vi "Main.vi"() -> ()   [LabVIEW 2017]
uses:
  <vilib>/LAVA/UI Tools/Fading/_Fade In(I32)__lava_lib_ui_tools.vi
  <vilib>/LAVA/UI Tools/Fading/_Fade Out(I32)__lava_lib_ui_tools.vi
panel:
  out "date string":string
  out "time string":string
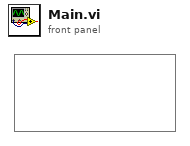
[diagram p1: front panel]
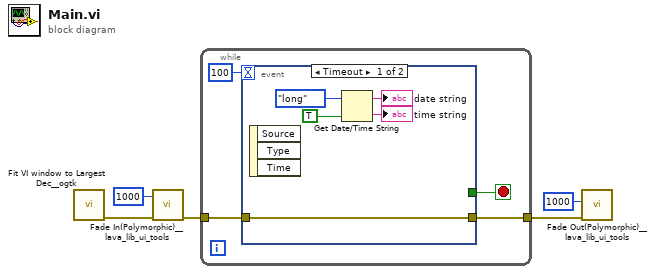
[diagram p0: block diagram]
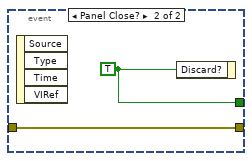
[diagram p2: hidden frame]
diagram:
  n1 = call <userlib>:"Fit VI window to Largest Dec__ogtk.vi"() -> ("error out"=w5:errorcluster)  [unwired: 6 in, 1 out]
  n2 = call-poly <vilib>:"Fade In(Polymorphic)__lava_lib_ui_tools.vi"("error in"=w5, "Fade time (ms)"=1000) -> ("error out"=w4:errorcluster)  [unwired: 8 in, 1 out]
  n3 = while {
    tunnel: w4 -> [w7]
    tunnel: [w6] -> w3
    stop <- w9 stop-if-true
    n4 = event shown="[0] Timeout" {
      selector: _ -> [_ _]
      dyn-events: _ -> [_ _]
      timeout: 100 -> [_ _]
      tunnel: [_ w16] -> w9
      tunnel: w7 -> [w10 w15]
      tunnel: [w10 w15] -> w6
      event Timeout {
        n5 = event-data() -> ()  [unwired: 1 in, 3 out]
        n6 = Get Date/Time String(date format (0)=enum16{"short", "long", "abbreviated"}."long", want seconds? (F)=TRUE) -> (date string=→"date string":string, time string=→"time string":string)  [unwired: 1 in]
      }
      event Panel Close? {
        w16 = TRUE ("Discard?")
        n7 = event-data() -> ()  [unwired: 1 in, 4 out]
        n8 = event-data("Discard?"=w16) -> ()  [unwired: 1 in, 1 out]
      }
    }
  }
  n9 = call-poly <vilib>:"Fade Out(Polymorphic)__lava_lib_ui_tools.vi"("error in"=w3, "Fade time (ms)"=1000) -> ()  [unwired: 8 in, 2 out]
